vi "Traffic lights.vi"() -> ()   [LabVIEW 2021]
panel:
  out "Blue":bool
  out "Green":bool
  out "Yellow":bool
  out "Red":bool
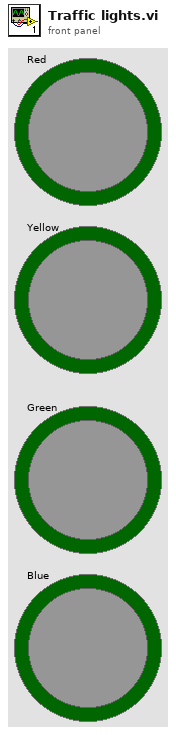
[diagram p1: front panel]
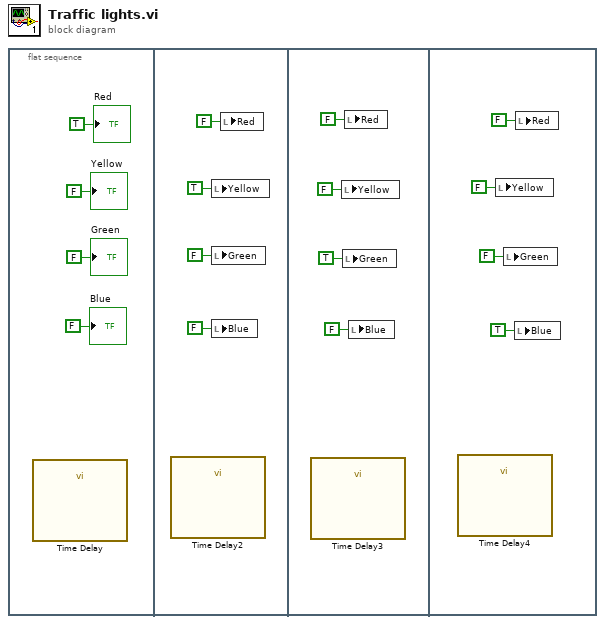
[diagram p0: block diagram]
diagram:
  n1 = flat-sequence {
    frame #0 {
      n2 = call "Time Delay"() -> ()  [unwired: 11 in, 1 out]
      "Red" <- TRUE ("Red")
      "Yellow" <- FALSE ("Yellow")
      "Green" <- FALSE ("Green")
      "Blue" <- FALSE ("Blue")
    }
    frame #1 {
      n3 = call "Time Delay2"() -> ()  [unwired: 11 in, 1 out]
      n4 = local write "Yellow"(TRUE ("Yellow")) -> ()
      n5 = local write "Green"(FALSE ("Green")) -> ()
      n6 = local write "Blue"(FALSE ("Blue")) -> ()
      n7 = local write "Red"(FALSE ("Red")) -> ()
    }
    frame #2 {
      n8 = call "Time Delay3"() -> ()  [unwired: 11 in, 1 out]
      n9 = local write "Yellow"(FALSE ("Yellow")) -> ()
      n10 = local write "Green"(TRUE ("Green")) -> ()
      n11 = local write "Red"(FALSE ("Red")) -> ()
      n12 = local write "Blue"(FALSE ("Blue")) -> ()
    }
    frame #3 {
      n13 = call "Time Delay4"() -> ()  [unwired: 11 in, 1 out]
      n14 = local write "Yellow"(FALSE ("Yellow")) -> ()
      n15 = local write "Green"(FALSE ("Green")) -> ()
      n16 = local write "Blue"(TRUE ("Blue")) -> ()
      n17 = local write "Red"(FALSE ("Red")) -> ()
    }
  }
